vi "filtraseriale (SubVI).vi"(8 "y":i32=290, 11 "angolo":i32) -> (3 "Boolean":bool)   [LabVIEW 2017]
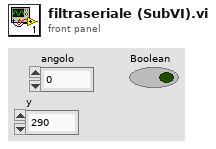
[diagram p1: front panel]
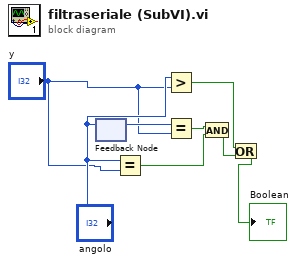
[diagram p0: block diagram]
diagram:
  n1 = feedback #1() -> (w2:i32)  [unwired: 1 in]
  n2 = feedback-in #1("angolo") -> ()
  n3 = Equal?(x="angolo", y="y") -> (x = y?=w5:bool)
  n4 = Greater?(x="angolo", y="y") -> (0:w8:bool)
  n5 = Equal?(x=w2, y="y") -> (x = y?=w4:bool)
  n6 = And(x=w4, y=w5) -> (x .and. y?=w7:bool)
  n7 = Or(x=w8, y=w7) -> (x .or. y?=→"Boolean":bool)
